vi "Autos Off.vi"(2 "error in":errorcluster, 4 "Targets":T1[](array[typedef]), 5 "queue in":refnum<queue>) -> (0 "error out":errorcluster, 1 "queue out":refnum<queue>)   [LabVIEW 2009]
uses:
  MixedMode/Messages/Mixed Mode Gui Update Msg.ctl
  MixedMode/Messages/Mixed Mode GUI Update Type.ctl
  MixedMode/Messages/Target.ctl
  Data Access Objects/Metadata/LBCB Number.ctl
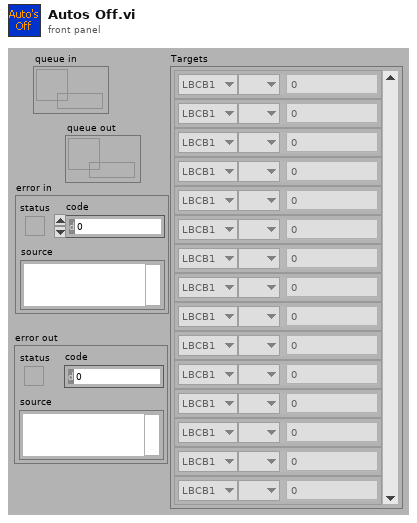
[diagram p1: front panel]
types:
  T1 = typedef "Target.ctl" = cluster{"LBCB Number":T2, "DOF Vectors":enum16{" ", "Dx", "Dy", "Dz", "Rx", "Ry", "Rz", "Fx", "Fy", "Fz", "Mx", "My", "Mz"}, "Amount":dbl}
  T2 = typedef "LBCB Number.ctl" = enum16{"LBCB1", "LBCB2"}
  T3 = typedef "Mixed Mode Gui Update Msg.ctl" = cluster{"MM GUI Update Type":T4, "Targets":T1[], "State":bool, "Step":string}
  T4 = typedef "Mixed Mode GUI Update Type.ctl" = enum16{"Nop", "Targets", "Accept.Blink", "Start.Blink", "TestStats", "Control.Enabled", "StartTestTimer", "RunInputFile", "NTCP Server", "Propose.Auto", "Execute.Auto", "All Autos Off", "Input File Loaded", "Exit"}
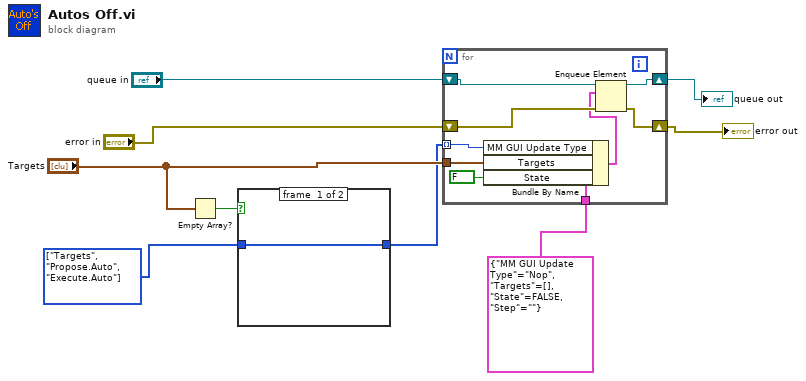
[diagram p0: block diagram]
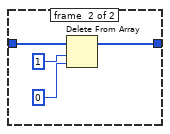
[diagram p2: hidden frame]
diagram:
  w2 = T4[] [enum."Targets", enum."Propose.Auto", enum."Execute.Auto"] items=["Nop", "Targets", "Accept.Blink", "Start.Blink", "TestStats", "Control.Enabled", "StartTestTimer", "RunInputFile", "NTCP Server", "Propose.Auto", "Execute.Auto", "All Autos Off", "Input File Loaded", "Exit"]
  n1 = Empty Array?(array="Targets") -> (empty?=w4:bool)
  n2 = case shown="True" w4 {
    tunnel: w2 -> [w10 w14]
    tunnel: [w10 w11] -> w1
    frame #0 {
    }
    frame #1 {
      n3 = Delete From Array(array=w14, length=1, index=0) -> (array with subset deleted=w11:T4[])  [unwired: 1 out]
    }
  }
  n4 = for {
    tunnel: T3 {"MM GUI Update Type"=enum."Nop", "Targets"=[], "State"=FALSE, "Step"=""} ("MM Gui Update Msg") -> [w21]
    tunnel: "Targets" -> [w19]
    tunnel: w1 -> [w18] mode=indexing
    shift-right: [w16] -> w9
    shift-left: "queue in" -> [w23]
    shift-right: [w17] -> w8
    shift-left: "error in" -> [w22]
    n5 = Bundle By Name(cluster=w21, "MM GUI Update Type"=w18, "Targets"=w19, "State"=FALSE) -> (w20:T3)
    n6 = Enqueue Element(queue=w23, element=w20, error in (no error)=w22) -> (queue out=w16:refnum<queue>, error out=w17:errorcluster)  [unwired: 1 in, 1 out]
  }
  "queue out" <- w9
  "error out" <- w8
